vi "Random Bitstream.vi"(0 "DataLen":i32) -> (1 "Array Size":i32, 2 "Array":i32[](array[numeric]))   [LabVIEW 2018]
doc: "Generates a Random Binary Stream of length DataLen"
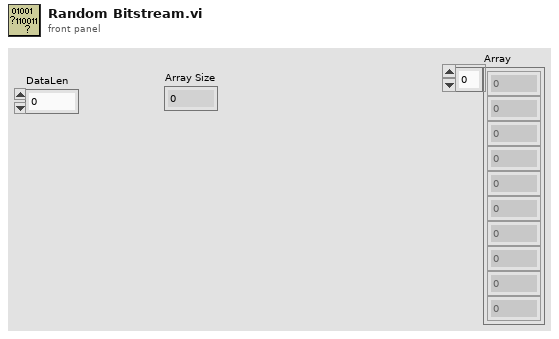
[diagram p1: front panel]
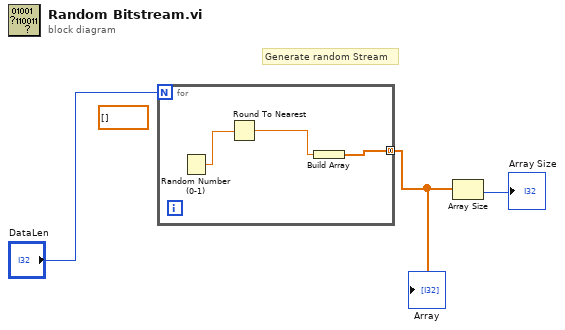
[diagram p0: block diagram]
diagram:
  (unwired) dbl[] []
  # "Generate random Stream"
  n1 = for {
    N: "DataLen" -> [_]
    tunnel: [w4] -> w3 mode=concatenating
    n2 = Random Number (0-1)() -> (number: 0 to 1=w6:dbl)
    n3 = Round To Nearest(number=w6) -> (nearest integer value=w5:dbl)
    n4 = Build Array(w5) -> (w4:dbl[])
  }
  "Array" <- w3
  n5 = Array Size(array=w3) -> (size(s)=→"Array Size":i32)
